vi "Layout - Read Panel Infos from Config.vi"(8 "error in (no error)":errorcluster) -> (0 "error out":errorcluster, 2 "Modules to load":string[](array[string]), 3 "Subpanel Labels":string[](array[string]))   [LabVIEW 2020, in "UI Manager.lvlib"]
doc: "Reads the subpanel labels and module names from the [panels] section of the UI Manager's configuration file and returns them.\n\n____\nHAMPEL SOFTWARE ENGINEERING v2.6.0 (2023-12-19 10:54)"
uses:
  UI Manager.lvlib
  Libraries/hse-libraries/Source/hse-application/hse-application.lvclass/hse-application.ctl
  Libraries/hse-libraries/Source/hse-application/HSE Application not initialized--error.vi
  <vilib>/Utility/error.llb/Clear Errors.vi
  Libraries/hse-libraries/Source/hse-application/hse-application__GetSingleton.vi
  <vilib>/Utility/sysdir.llb/Get System Directory.vi
  <vilib>/Utility/error.llb/Error Cluster From Error Code.vi
  <vilib>/Utility/config.llb/Read Key (String).vi
  Libraries/hse-libraries/Source/hse-application/hse-application.lvclass
  <vilib>/Utility/config.llb/NI_LVConfig.lvlib
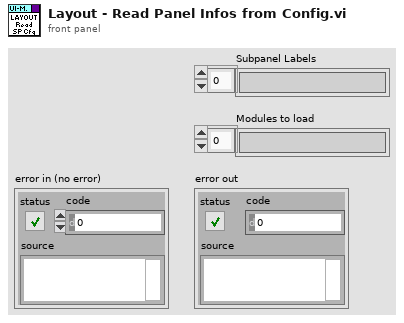
[diagram p1: front panel]
types:
  T1 = typedef "NI_LVConfig.lvlib/Config Data RefNum.ctl" = refnum<k1>
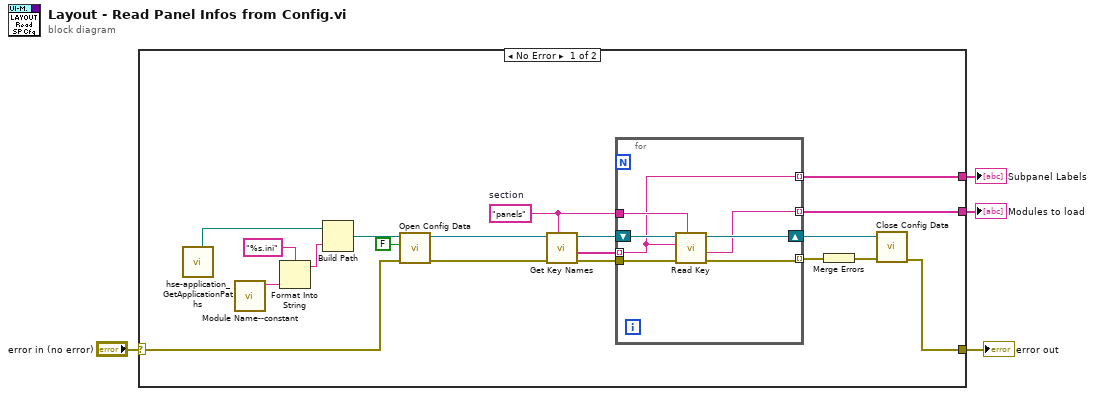
[diagram p0: block diagram]
diagram:
  n1 = case shown="No Error" "error in (no error)" {
    selector: "error in (no error)" -> [w17 w31]
    tunnel: [w7 w31] -> w3
    tunnel: [w6 _] -> w2
    tunnel: [w5 _] -> w1
    frame No Error {
      w11 = "panels"  # section
      n2 = call "hse-application_GetApplicationPaths.vi"() -> ("Config/Unit Directory"=w21:path)  [unwired: 5 in, 6 out]
      n3 = call "Module Name--constant.vi"() -> ("Module Name"=w20:string)  [unwired: 11 in]
      n4 = Format Into String(format string="%s.ini", w20) -> (resulting string=w22:string)  [unwired: 2 in, 1 out]
      n5 = Build Path(base path=w21, name or relative path=w22) -> (appended path=w18:path)
      n6 = call <vilib>:"Open Config Data.vi"("error in (no error)"=w17, "create file if necessary (T)"=FALSE, "configuration file path"=w18) -> ("error out"=w15:errorcluster, "refnum"=w16:T1)  [unwired: 6 in, 1 out]
      n7 = call <vilib>:"Get Key Names.vi"("section"=w11, "error in (no error)"=w15, "refnum"=w16) -> ("error out"=w13:errorcluster, "key names"=w12:string[], "refnum out"=w14:T1)  [unwired: 5 in, 1 out]
      n8 = for {
        tunnel: w13 -> [w29]
        tunnel: w12 -> [w25] mode=indexing
        tunnel: w11 -> [w28]
        shift-right: [w27] -> w10
        shift-left: w14 -> [w30]
        tunnel: [w26] -> w9 mode=indexing
        tunnel: [w25] -> w6 mode=indexing
        tunnel: [w24] -> w5 mode=indexing
        n9 = call-poly <vilib>:"Read Key.vi"("section"=w28, "error in (no error)"=w29, "key"=w25, "refnum"=w30) -> ("error out"=w26:errorcluster, "value"=w24:string, "refnum out"=w27:T1)  [unwired: 4 in, 1 out]
      }
      n10 = Merge Errors(w9) -> (w8:errorcluster)
      n11 = call <vilib>:"Close Config Data.vi"("error in (no error)"=w8, "refnum"=w10) -> ("error out"=w7:errorcluster)  [unwired: 8 in, 1 out]
    }
    frame Error {
    }
  }
  "error out" <- w3
  "Subpanel Labels" <- w2
  "Modules to load" <- w1
